vi "Detect Infinite Pattern.vi"(7 "Positon Grid":T1[][](array[typedef]), 8 "Start Direction":T2, 10 "Start Position":T1, 11 "Grid":string[][](array[string])) -> (3 "Infinite Detected Out":bool)   [LabVIEW 2024]
uses:
  Cluster_Position.ctl
  ENUM_Direction.ctl
panel:
  out "Numeric":i32
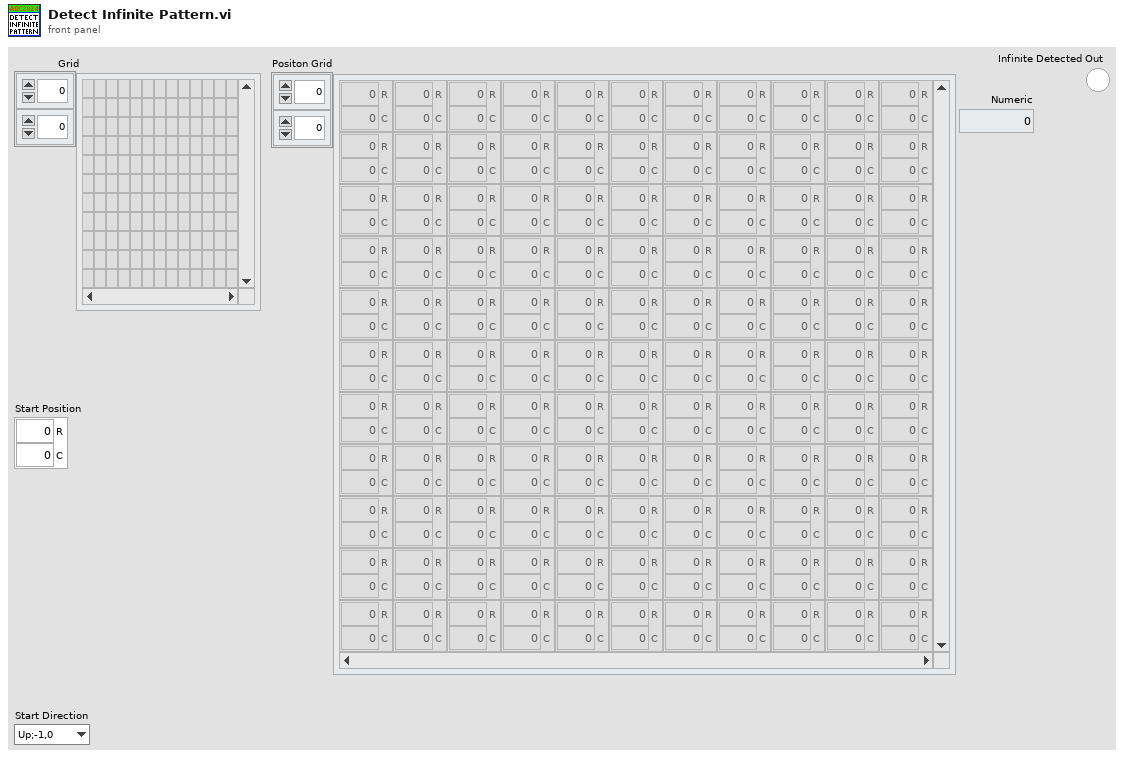
[diagram p1: front panel]
types:
  T1 = typedef "Cluster_Position.ctl" = cluster{"R":i32, "C":i32}
  T2 = typedef "ENUM_Direction.ctl" = enum16{"Up;-1,0", "Right;0,1", "Down;1,0", "Left;0,-1"}
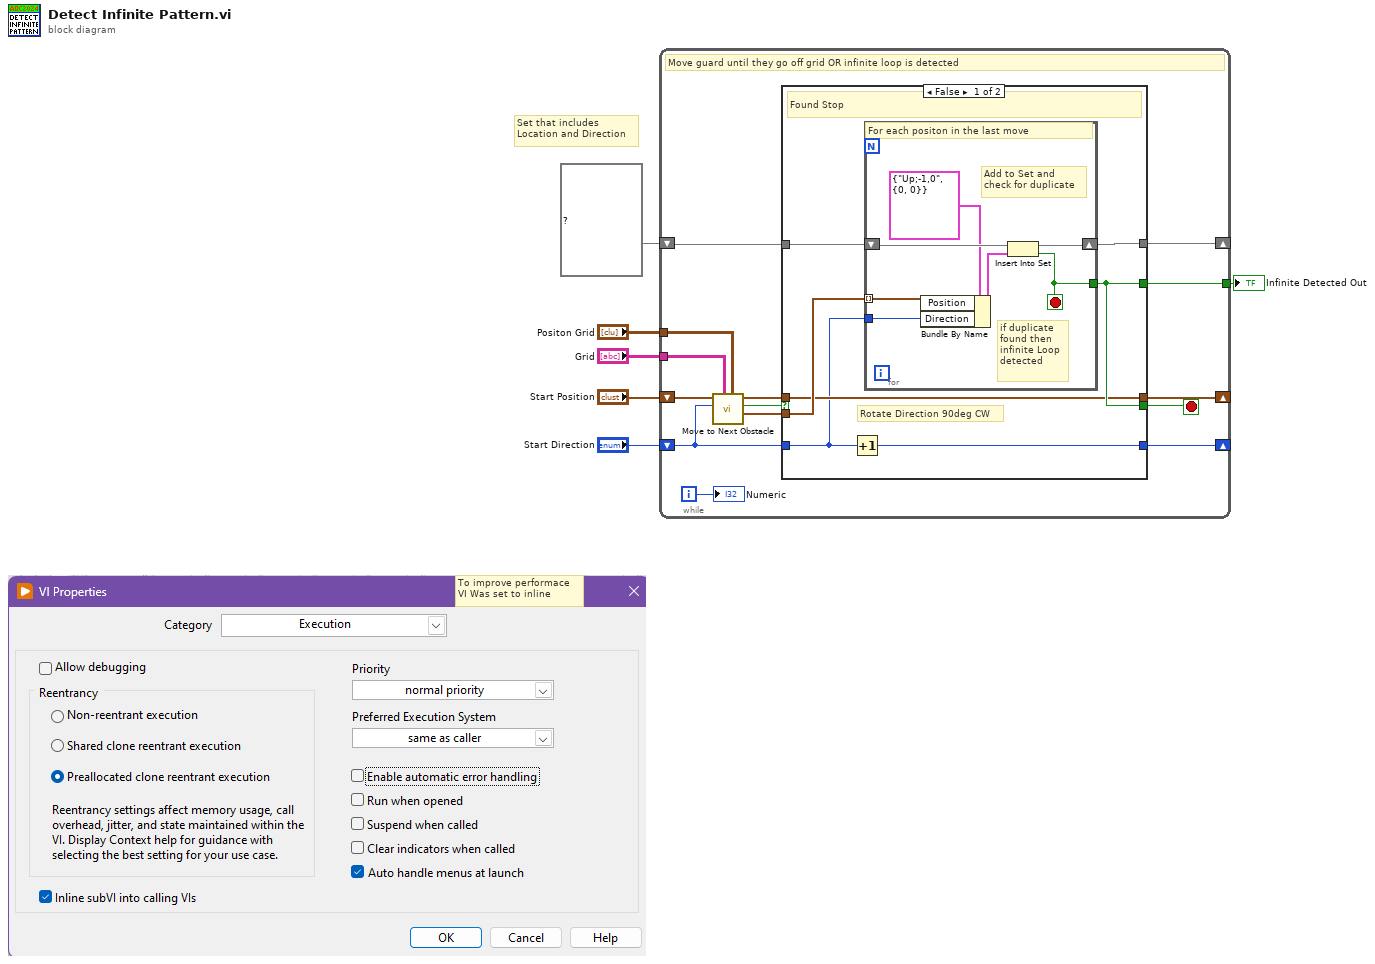
[diagram p0: block diagram]
diagram:
  # "To improve performace\nVI Was set to inline"
  # "Set that includes\nLocation and Direction"
  n1 = while {
    tunnel: "Grid" -> [w9]
    shift-right: [w12] -> _
    shift-left: "Start Position" -> [w8]
    shift-right: [w11] -> _
    shift-left: "Start Direction" -> [w18]
    shift-right: [w17] -> _
    shift-left: set{cluster{"Direction":T2, "Position":T1}} {} ("Set") -> [w20]
    tunnel: [w13] -> w6
    tunnel: "Positon Grid" -> [w10]
    i -> [w7]
    stop <- w16 stop-if-true
    # "Move guard until they go off grid OR infinite loop is detected"
    n2 = call "Move to Next Obstacle.vi"("Positon Grid"=w10, "Grid"=w9, "Direction"=w18, "Start Postion"=w8) -> ("Positions Covered Out"=w19:T1[], "OFF Grid Out"=w15:bool, "End Position Out"=w14:T1)  [unwired: 5 in]
    n3 = case shown="False" w15 {
      selector: w15 -> [_ w37]
      tunnel: w20 -> [w27 w38]
      tunnel: w19 -> [w26 _]
      tunnel: w18 -> [w22 w35]
      tunnel: [w25 w38] -> w17
      tunnel: [w24 w37] -> w16
      tunnel: w14 -> [w23 w36]
      tunnel: [w24 _] -> w13
      tunnel: [w23 w36] -> w12
      tunnel: [w21 w35] -> w11
      frame False {
        # "Rotate Direction 90deg CW"
        # "Found Stop"
        n4 = Increment(x=w22) -> (x+1=w21:T2)
        n5 = for {
          shift-right: [w33] -> w25
          shift-left: w27 -> [w34]
          tunnel: w26 -> [w30] mode=indexing
          tunnel: w22 -> [w29]
          tunnel: [w28] -> w24
          stop <- w28 stop-if-true
          # "if duplicate\nfound then\ninfinite Loop\ndetected"
          # "Add to Set and \ncheck for duplicate"
          # "For each positon in the last move"
          n6 = Bundle By Name(cluster=cluster{"Direction":T2, "Position":T1} {"Direction"=enum."Up;-1,0", "Position"={"R"=0, "C"=0}} ("element"), "Position"=w30, "Direction"=w29) -> (w31:cluster{"Direction":T2, "Position":T1})
          n7 = Insert Into Set(10:w31, 11:w34) -> (2:w28:bool, 3:w33:set{cluster{"Direction":T2, "Position":T1}})
        }
      }
      frame True {
        # "OFF Grid"
      }
    }
    "Numeric" <- w7
  }
  "Infinite Detected Out" <- w6
